vi "EXCOM-26.vi"(0 "VRN IN":refnum<visa-resource-name>, 1 "Bool Refnum":refnum<vi>, 11 "Error IN":errorcluster) -> (2 "STATL":bool[](array[boolean])=[TRUE, FALSE, FALSE, FALSE, FALSE, FALSE, FALSE, FALSE, FALSE, FALSE, FALSE, FALSE, FALSE, FALSE, FALSE, FALSE, FALSE, FALSE, FALSE, FALSE, FALSE, FALSE, FALSE, FALSE, FALSE, FALSE, FALSE, FALSE, FALSE, FALSE, FALSE, FALSE], 3 "STATH":bool[](array[boolean])=[FALSE, FALSE, TRUE, TRUE, FALSE, TRUE, TRUE, FALSE, FALSE, FALSE, FALSE, FALSE, FALSE, FALSE, FALSE, FALSE, FALSE, FALSE, FALSE, FALSE, FALSE, FALSE, FALSE, FALSE, FALSE, FALSE, FALSE, FALSE, FALSE, FALSE, FALSE, FALSE], 4 "VRN OUT":refnum<visa-resource-name>, 8 "OK Done":bool=TRUE, 13 "STATEX":bool[](array[boolean]), 14 "STATLH":bool[](array[boolean]), 15 "Error OUT":errorcluster)   [LabVIEW 2019]
panel:
  out "Answer":string
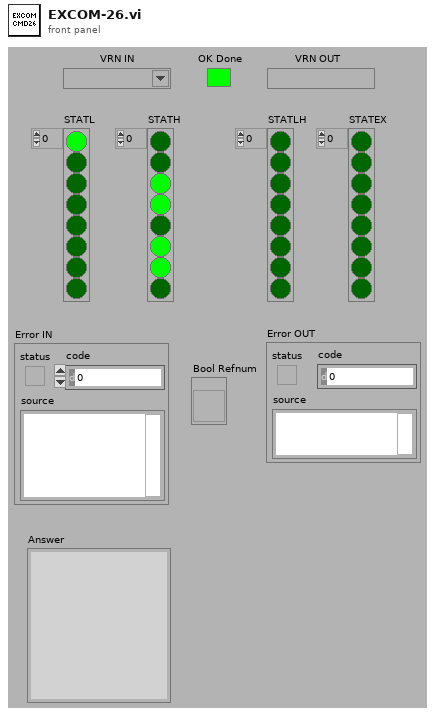
[diagram p1: front panel]
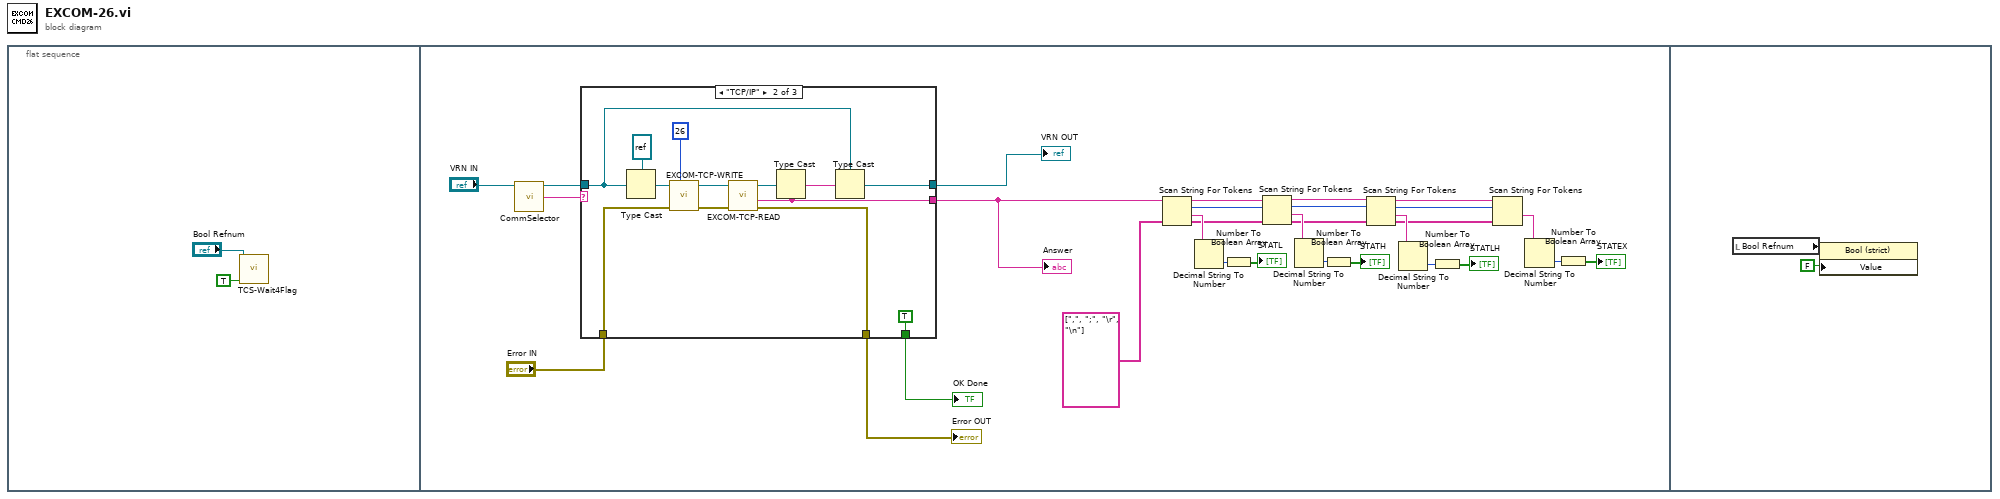
[diagram p0: block diagram]
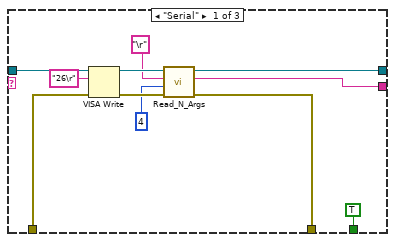
[diagram p2: hidden frame]
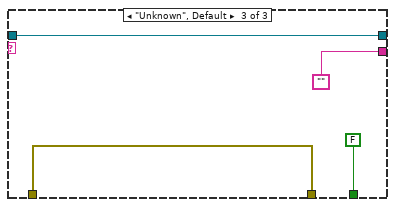
[diagram p3: hidden frame]
diagram:
  n1 = flat-sequence {
    frame #0 {
      n2 = call "TCS-Wait4Flag.vi"("Raise Flag ?"=TRUE, "Ctl Refnum IN"="Bool Refnum") -> ()  [unwired: 8 in, 2 out]
    }
    frame #1 {
      w3 = string[] [",", ";", "\r", "\n"] ("delimiters (\\s,\\t,\\r,\\n)")
      n3 = call "CommSelector.vi"("VISA resource name"="VRN IN") -> ("VISA resource name"=w7:refnum<visa-resource-name>, "CommType"=w6:string)  [unwired: 13 in]
      n4 = case shown="\"TCP/IP\"" w6 {
        tunnel: [w34 w42 w55] -> w29
        tunnel: [w36 w41 w56] -> w28
        tunnel: [TRUE ("status") TRUE ("status") FALSE ("status")] -> w27
        tunnel: "Error IN" -> [w33 w47 w56]
        tunnel: w7 -> [w31 w43 w55]
        tunnel: [w30 w45 ""] -> w4
        frame "Serial" {
          n5 = VISA Write(VISA resource name=w31, write buffer="26\r" ("String to Send"), error in (no error)=w33) -> (VISA resource name out=w39:refnum<visa-resource-name>, error out=w40:errorcluster)  [unwired: 1 out]
          n6 = call "Read_N_Args.vi"("Error IN"=w40, "Nb_Args"=4, "Arg_Char"="\r", "VRN IN"=w39) -> ("Error OUT"=w36:errorcluster, "Answer"=w30:string, "VRN OUT"=w34:refnum<visa-resource-name>)  [unwired: 4 in, 1 out]
        }
        frame "TCP/IP" {
          n7 = Type Cast(type=refnum<k5> refnum ("connection ID"), x=w43) -> (*(type *) &x=w48:refnum<k5>)
          n8 = call "EXCOM-TCP-WRITE.vi"("Commande #"=26, "Error IN"=w47, "connection ID"=w48) -> ("Error OUT"=w52:errorcluster, "connection ID out"=w51:refnum<k5>)  [unwired: 4 in, 2 out]
          n9 = call "EXCOM-TCP-READ.vi"("Error In"=w52, "connection ID"=w51) -> ("Error Out"=w41:errorcluster, "Response"=w45:string, "CID Out"=w46:refnum<k5>)  [unwired: 5 in]
          n10 = Type Cast(type=w45, x=w46) -> (*(type *) &x=w44:string)
          n11 = Type Cast(type=w43, x=w44) -> (*(type *) &x=w42:refnum<visa-resource-name>)
        }
        frame "Unknown", Default {
        }
      }
      "VRN OUT" <- w29
      "Error OUT" <- w28
      "OK Done" <- w27
      "Answer" <- w4
      n12 = Scan String For Tokens(6:w3, 9:w4) -> (1:w8:string, 2:w13:i32, 3:w11:string)  [unwired: 4 in, 1 out]
      n13 = Decimal String To Number(string=w8) -> (number=w15:i32)  [unwired: 2 in, 1 out]
      n14 = Number To Boolean Array(number=w15) -> (Boolean array=→"STATL":bool[])
      n15 = Scan String For Tokens(6:w3, 8:w13, 9:w11) -> (1:w9:string, 2:w14:i32, 3:w12:string)  [unwired: 3 in, 1 out]
      n16 = Decimal String To Number(string=w9) -> (number=w17:i32)  [unwired: 2 in, 1 out]
      n17 = Number To Boolean Array(number=w17) -> (Boolean array=→"STATH":bool[])
      n18 = Scan String For Tokens(6:w3, 8:w14, 9:w12) -> (1:w10:string, 2:w23:i32, 3:w24:string)  [unwired: 3 in, 1 out]
      n19 = Decimal String To Number(string=w10) -> (number=w18:i32)  [unwired: 2 in, 1 out]
      n20 = Number To Boolean Array(number=w18) -> (Boolean array=→"STATLH":bool[])
      n21 = Scan String For Tokens(6:w3, 8:w23, 9:w24) -> (1:w21:string)  [unwired: 3 in, 3 out]
      n22 = Decimal String To Number(string=w21) -> (number=w22:i32)  [unwired: 2 in, 1 out]
      n23 = Number To Boolean Array(number=w22) -> (Boolean array=→"STATEX":bool[])
    }
    frame #2 {
      n24 = local read "Bool Refnum"() -> (w58:refnum<vi>)
      n25 = property on="Property Node" class="Bool (strict)"(reference=w58, "Value"=FALSE) -> ()  [unwired: 1 in, 2 out]
    }
  }
